vi "标准存取.vi"() -> ()   [LabVIEW 2018]
panel:
  out "文本 2":string[](array[string])
  in  "计数":i32
  in  "文本":string
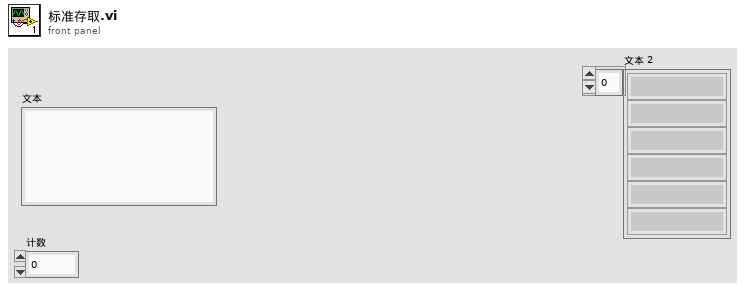
[diagram p1: front panel]
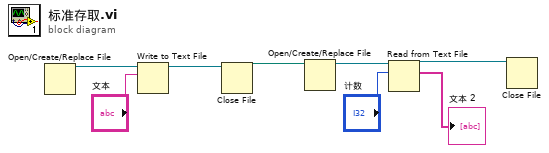
[diagram p0: block diagram]
diagram:
  n1 = Open/Create/Replace File() -> (refnum out=w8:refnum<file>)  [unwired: 6 in, 2 out]
  n2 = Write to Text File(file (use dialog)=w8, text="文本") -> (refnum out=w6:refnum<file>)  [unwired: 2 in, 2 out]
  n3 = Close File(refnum=w6) -> (path=w5:path)  [unwired: 1 in, 1 out]
  n4 = Open/Create/Replace File(file path (use dialog)=w5) -> (refnum out=w4:refnum<file>)  [unwired: 5 in, 2 out]
  n5 = Read from Text File(file (use dialog)=w4, count="计数") -> (refnum out=w2:refnum<file>, text=→"文本 2":string[])  [unwired: 2 in, 2 out]
  n6 = Close File(refnum=w2) -> ()  [unwired: 1 in, 2 out]
